vi "XY error bars_diag.vi"(1 "XY plot":cluster{dbl[], dbl[]}(graph), 2 "Xerror":dbl[](array[numeric]), 3 "Yerror":dbl[](array[numeric])) -> (4 "X+Y error bars":cluster{dbl[], dbl[]}(graph), 5 "Y error bars":cluster{dbl[], dbl[]}(graph), 6 "X error bars":cluster{dbl[], dbl[]}(graph))   [LabVIEW 2015]
doc: "This VI allows for the addition of error bars to a XY scatter plot in X, Y or both directions.\n\nThe mandatory XY plot input should contain the plot to which error bars are to be added; the Xerror and Yerror inputs contain the point by point error in these scatter plot points.\n\nThe outputs are in the XY scatter plot data type, which can readily be appended to an existing plot.\n\n\n© 2007, VU University Amsterdam\nJoost van Mameren, jmameren@gmail.com"
panel:
  in  "?":T1(tab)
  # "© 2007 VU University, Amsterdam\nJoost van Mameren, jmameren@gmail.com"
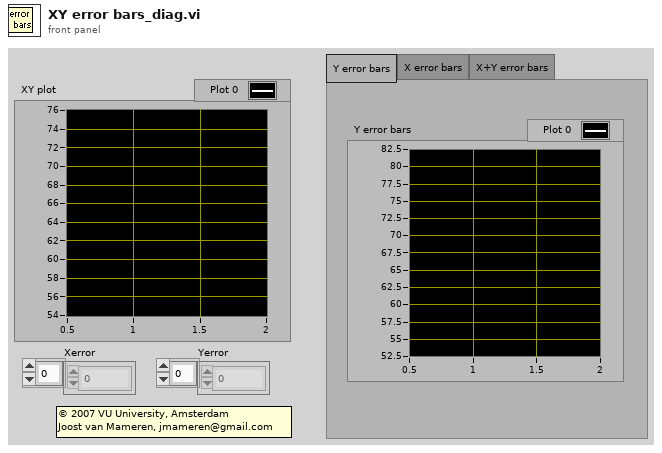
[diagram p1: front panel]
types:
  T1 = enum32{"Y error bars", "X error bars", "X+Y error bars"}
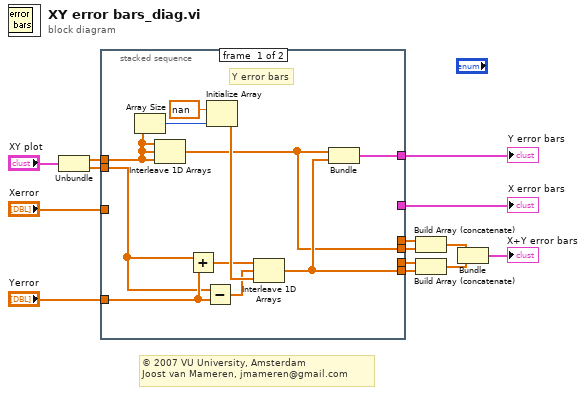
[diagram p0: block diagram]
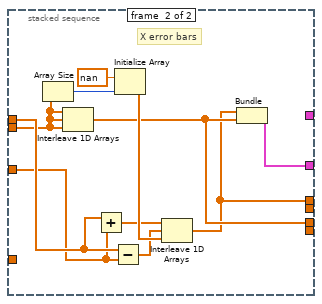
[diagram p2: hidden frame]
diagram:
  # "© 2007 VU University, Amsterdam\nJoost van Mameren, jmameren@gmail.com"
  n1 = Unbundle("XY plot") -> (w2:dbl[], w1:dbl[])
  n2 = stacked-sequence {
    tunnel: w1 -> [w15 w29]
    tunnel: w2 -> [w20 w30]
    tunnel: "Yerror" -> [w18 _]
    tunnel: [w19 _] -> w12
    tunnel: [_ w31] -> w11
    tunnel: "Xerror" -> [_ w28]
    tunnel: [_ w27] -> w10
    tunnel: [w17 _] -> w9
    tunnel: [w16 _] -> w6
    tunnel: [_ w26] -> w5
    frame #0 {
      # "Y error bars"
      n3 = Array Size(array=w20) -> (size(s)=w23:i32)
      n4 = Interleave 1D Arrays(w20, w20, w20) -> (w16:dbl[])
      n5 = Add(x=w15, y=w18) -> (x+y=w21:dbl[])
      n6 = Subtract(x=w15, y=w18) -> (x-y=w22:dbl[])
      n7 = Initialize Array(nan ("element"), w23) -> (w24:dbl[])
      n8 = Interleave 1D Arrays(w21, w22, w24) -> (w17:dbl[])
      n9 = Bundle(w16, w17) -> (w19:cluster{dbl[], dbl[]})  [unwired: 1 in]
    }
    frame #1 {
      # "X error bars"
      n10 = Array Size(array=w29) -> (size(s)=w34:i32)
      n11 = Interleave 1D Arrays(w29, w29, w29) -> (w27:dbl[])
      n12 = Add(x=w30, y=w28) -> (x+y=w32:dbl[])
      n13 = Subtract(x=w30, y=w28) -> (x-y=w33:dbl[])
      n14 = Initialize Array(nan ("element"), w34) -> (w35:dbl[])
      n15 = Interleave 1D Arrays(w32, w33, w35) -> (w26:dbl[])
      n16 = Bundle(w26, w27) -> (w31:cluster{dbl[], dbl[]})  [unwired: 1 in]
    }
  }
  "X error bars" <- w11
  "Y error bars" <- w12
  n17 = Build Array (concatenate)(w5, w6) -> (w7:dbl[])
  n18 = Build Array (concatenate)(w10, w9) -> (w8:dbl[])
  n19 = Bundle(w7, w8) -> (→"X+Y error bars":cluster{dbl[], dbl[]})  [unwired: 1 in]
